vi "unused_Read ref.vi"(8 "error in (no error)":errorcluster, 11 "GObject in":refnum<class "GObject.lvclass">) -> (0 "error out":errorcluster, 2 "ref":refnum<vi>, 3 "GObject out":refnum<class "GObject.lvclass">)   [LabVIEW 2023]
uses:
  GObject.lvclass/GObject.ctl
  GObject.lvclass
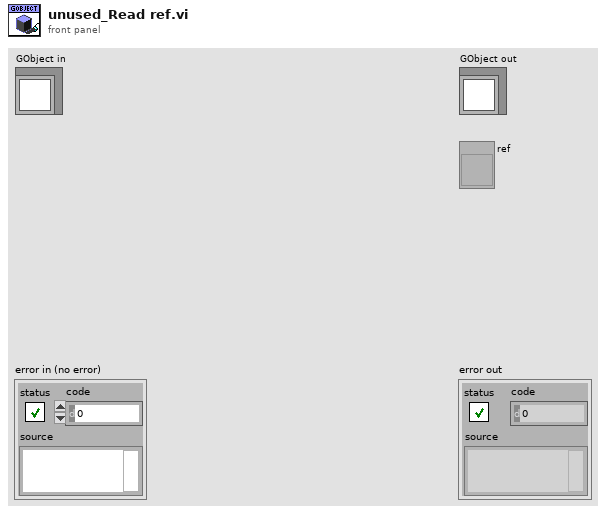
[diagram p1: front panel]
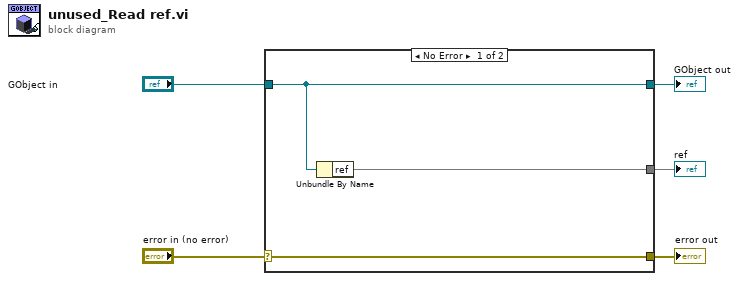
[diagram p0: block diagram]
diagram:
  n1 = case shown="No Error" "error in (no error)" {
    selector: "error in (no error)" -> [w8 w9]
    tunnel: [w8 w9] -> w4
    tunnel: [w7 w10] -> w2
    tunnel: "GObject in" -> [w7 w10]
    tunnel: [w6 _] -> w1
    frame No Error {
      n2 = Unbundle By Name(w7) -> ("ref"=w6)
    }
    frame Error {
    }
  }
  "error out" <- w4
  "GObject out" <- w2
  "ref" <- w1
